vi "git_push.vi"(11 "Working Dir":path) -> ()   [LabVIEW 2020, in "AJ_QuickDrop_Git.lvlib"]
uses:
  <resource>/dialog/QuickDrop/plugins/AJ_QD_Git/AJ_QuickDrop_Git.lvlib
  <vilib>/Hampel Software Engineering/Git API/Source/Git API/GIT-api.lvclass
panel:
  out "Working Directory":path
  in  "Cancel":bool
  in  "Add":bool
  out "Git Log":string="Committed from LabVIEW Quick Drop"
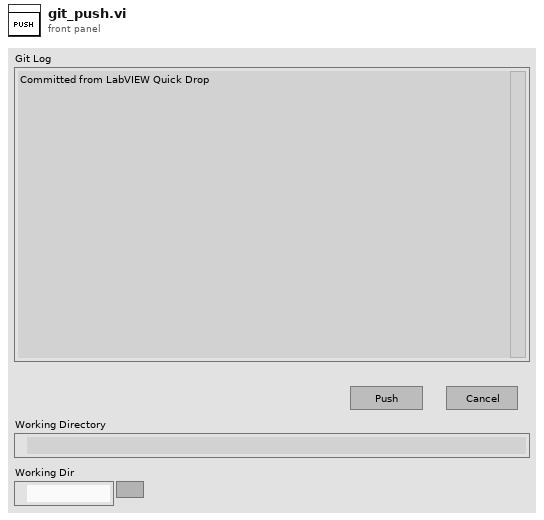
[diagram p1: front panel]
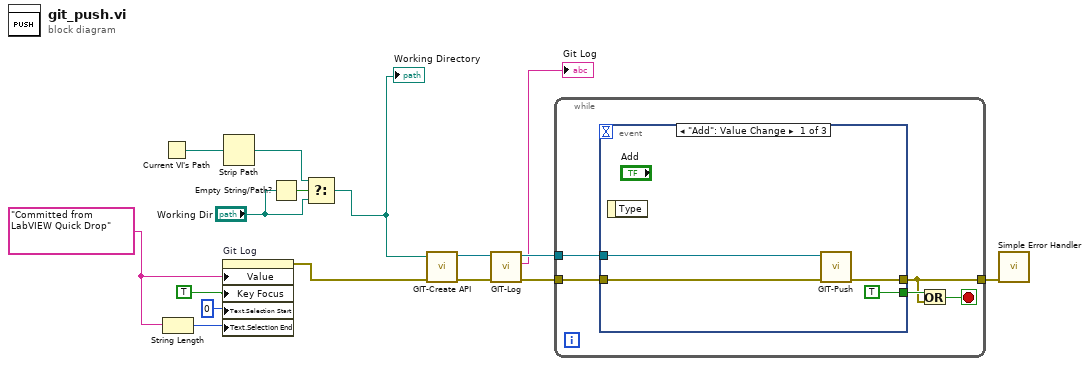
[diagram p0: block diagram]
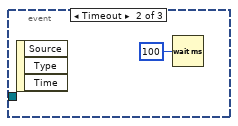
[diagram p2: hidden frame]
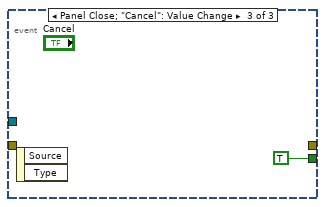
[diagram p3: hidden frame]
diagram:
  w14 = "Committed from LabVIEW Quick Drop" ("Commit Message")
  n1 = Current VI's Path() -> (path=w10:path)
  n2 = String Length(string=w14) -> (length=w13:i32)
  n3 = property on="Git Log" class="Str"("Value"=w14, "Key Focus"=TRUE, "Text.Selection Start"=u32 0 ("Text.Selection:Start"), "Text.Selection End"=w13) -> (error out=w5:errorcluster)  [unwired: 2 in, 1 out]
  n4 = Strip Path(path=w10) -> (stripped path=w8:path)  [unwired: 1 out]
  n5 = Empty String/Path?(string/path="Working Dir") -> (empty?=w11:bool)
  n6 = Select(t=w8, s=w11, f="Working Dir") -> (s? t:f=w6:path)
  "Working Directory" <- w6
  n7 = call <vilib>:"GIT-Create API.vi"("error in"=w5, "Working Dir"=w6) -> ("error out"=w2:errorcluster, "git-api out"=w7:refnum<class "GIT-api.lvclass">)  [unwired: 8 in]
  n8 = call <vilib>:"GIT-Log.vi"("error in"=w2, "git-api in"=w7) -> ("error out"=w1:errorcluster, "std out"=→"Git Log":string, "git-api out"=w4:refnum<class "GIT-api.lvclass">)  [unwired: 7 in]
  n9 = while {
    tunnel: [w19] -> w12
    tunnel: w1 -> [w18]
    tunnel: w4 -> [w17]
    stop <- w20 stop-if-true
    n10 = event shown="[0] \"Add\": Value Change" {
      selector: _ -> [_ _ _]
      dyn-events: _ -> [_ _ _]
      timeout: _ -> [_ _ _]
      tunnel: [TRUE _ TRUE] -> w21
      tunnel: [w25 _ _] -> w19
      tunnel: w18 -> [w22 _ _]
      tunnel: w17 -> [w23 _ _]
      event "Add": Value Change {
        n11 = event-data() -> ()  [unwired: 1 in, 1 out]
        n12 = call <vilib>:"GIT-Push.vi"("error in"=w22, "Git-API in"=w23) -> ("error out"=w25:errorcluster)  [unwired: 7 in, 2 out]
      }
      event Timeout {
        n13 = event-data() -> ()  [unwired: 1 in, 3 out]
        n14 = Wait (ms)(milliseconds to wait=u32 100) -> ()  [unwired: 1 out]
      }
      event Panel Close; "Cancel": Value Change {
        n15 = event-data() -> ()  [unwired: 1 in, 2 out]
      }
    }
    n16 = Or(x=w21, y=w19) -> (x .or. y?=w20:bool)
  }
  n17 = call <vilib>:"Simple Error Handler.vi"("error in (no error)"=w12) -> ()  [unwired: 4 in, 5 out]
